vi "Config Marker Destination.vi"(0 "VISA Resource Name":refnum<visa-resource-name>, 1 "Standard (0: IS-95A)":T1(ring), 2 "Pulse (0: NONE)":enum16{"NONE", "M1", "M2", "M3", "M4"}(ring), 3 "Alternate Amplitude (0: NONE)":enum16{"NONE", "M1", "M2", "M3", "M4"}(ring), 4 "ALC Hold (0: NONE)":enum16{"NONE", "M1", "M2", "M3", "M4"}(ring), 5 "error in (no error)":errorcluster {"code" format="%.0x"}) -> (14 "VISA Resource Name Out":refnum<visa-resource-name>, 19 "error out":errorcluster {"code" format="%.0x"})   [LabVIEW 2014, in "Agilent ESG Series.lvlib"]
doc: "This VI configures the I/Q modulation signals for CDMA arbitrary system.\n\nNotes:\n(1) This VI is valid only on instrument E4438C."
uses:
  Agilent ESG Series.lvlib
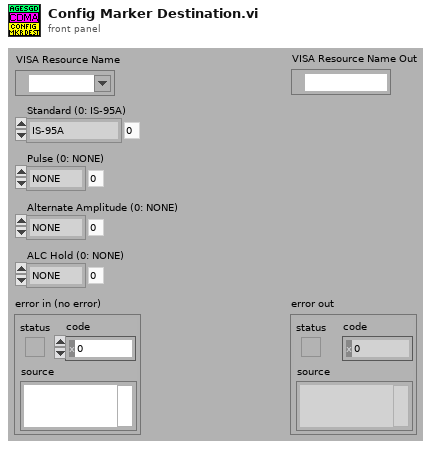
[diagram p1: front panel]
types:
  T1 = enum16{"IS-95A", "CDMA2000", "WCDMA", "Dual Arbitrary"}
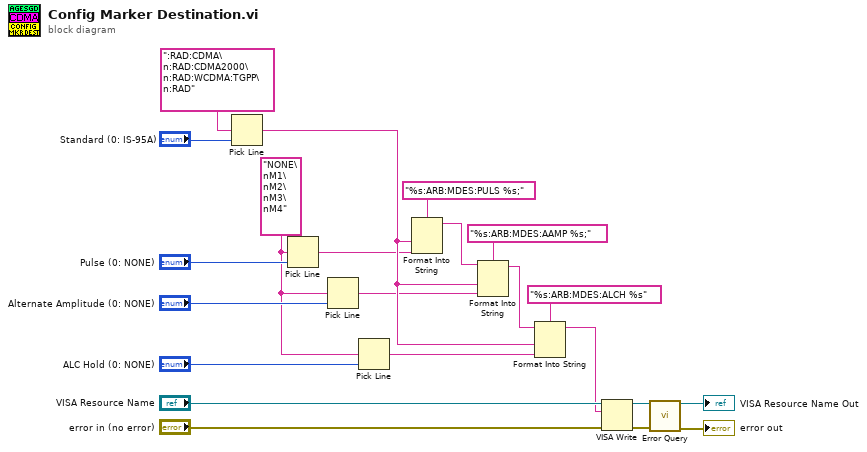
[diagram p0: block diagram]
diagram:
  w6 = "NONE\nM1\nM2\nM3\nM4"
  n1 = Pick Line(multi-line string=":RAD:CDMA\n:RAD:CDMA2000\n:RAD:WCDMA:TGPP\n:RAD", line index="Standard (0: IS-95A)") -> (output string=w14:string)  [unwired: 1 in]
  n2 = Pick Line(multi-line string=w6, line index="Pulse (0: NONE)") -> (output string=w5:string)  [unwired: 1 in]
  n3 = Pick Line(multi-line string=w6, line index="Alternate Amplitude (0: NONE)") -> (output string=w4:string)  [unwired: 1 in]
  n4 = Pick Line(multi-line string=w6, line index="ALC Hold (0: NONE)") -> (output string=w3:string)  [unwired: 1 in]
  n5 = Format Into String(format string="%s:ARB:MDES:PULS %s;", w14, w5) -> (resulting string=w11:string)  [unwired: 2 in, 1 out]
  n6 = Format Into String(format string="%s:ARB:MDES:AAMP %s;", initial string=w11, w14, w4) -> (resulting string=w10:string)  [unwired: 1 in, 1 out]
  n7 = Format Into String(format string="%s:ARB:MDES:ALCH %s", initial string=w10, w14, w3) -> (resulting string=w2:string)  [unwired: 1 in, 1 out]
  n8 = VISA Write(VISA resource name="VISA Resource Name", write buffer=w2, error in (no error)="error in (no error)") -> (VISA resource name out=w18:refnum<visa-resource-name>, error out=w17:errorcluster)  [unwired: 1 out]
  n9 = call "Error Query.vi"("VISA Resource Name"=w18, "error in (no error)"=w17) -> ("VISA Resource Name Out"=→"VISA Resource Name Out":refnum<visa-resource-name>, "error out"=→"error out":errorcluster)  [unwired: 10 in, 2 out]
